vi "PRL DW Check Data CSG.vi"(11 "Data":csg[](array[numeric])) -> (3 "Bad Data?":bool[](array[boolean]))   [LabVIEW 2018, in "S3DK.lvlib" / "PMU Recorder Light.lvlib"]
uses:
  PMU Recorder Light.lvlib
  Setting Choice.ctl
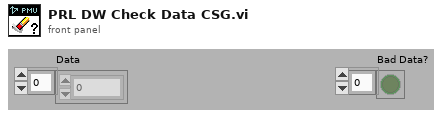
[diagram p1: front panel]
types:
  T1 = typedef "S3DK.lvlib/PMU Recorder Light.lvlib/Setting Choice.ctl" = enum16{"Analog Data Points Allowed Equals", "Complex Data Points Allowed Equals", "Seconds Before Reset After Wait for Config Fails", "Number of Live Buffer in Access Buffer ", "Number of Connection Attempts", "Live Data Buffer Size", "dt Tolerance", "Data Rate History", "ALL"}
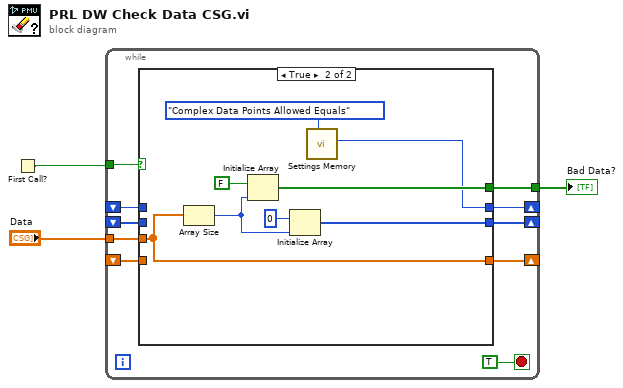
[diagram p0: block diagram]
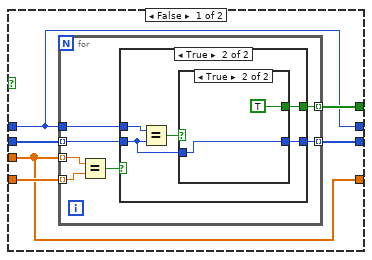
[diagram p2: hidden frame]
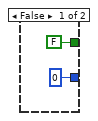
[diagram p3: hidden frame]
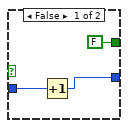
[diagram p4: hidden frame]
diagram:
  n1 = First Call?() -> (First Call?: T/F=w1:bool)
  n2 = while {
    tunnel: w1 -> [w13]
    tunnel: "Data" -> [w12]
    shift-right: [w10] -> _
    shift-left: _ -> [w7]
    shift-right: [w11] -> _
    shift-left: _ -> [w8]
    tunnel: [w9] -> w2
    shift-right: [w5] -> _
    shift-left: _ -> [w6]
    stop <- TRUE stop-if-true
    n3 = case shown="True" w13 {
      tunnel: w12 -> [w17 w44]
      tunnel: [w16 w45] -> w11
      tunnel: [w17 w44] -> w10
      tunnel: [w15 w41] -> w9
      tunnel: w8 -> [w19 _]
      tunnel: w7 -> [w18 _]
      tunnel: w6 -> [w14 _]
      tunnel: [w14 w39] -> w5
      frame False {
        n4 = for {
          tunnel: w19 -> [w23] mode=indexing
          tunnel: w17 -> [w25] mode=indexing
          tunnel: w18 -> [w26] mode=indexing
          tunnel: w14 -> [w22]
          tunnel: [w21] -> w16 mode=indexing
          tunnel: [w20] -> w15 mode=indexing
          n5 = Equal?(x=w25, y=w26) -> (x = y?=w24:bool)
          n6 = case shown="True" w24 {
            tunnel: w23 -> [_ w31]
            tunnel: w22 -> [_ w33]
            tunnel: [0 w30] -> w21
            tunnel: [FALSE w29] -> w20
            frame False {
            }
            frame True {
              n7 = Equal?(x=w33, y=w31) -> (x = y?=w32:bool)
              n8 = case shown="True" w32 {
                tunnel: w31 -> [w36 w38]
                tunnel: [w35 w38] -> w30
                tunnel: [FALSE TRUE] -> w29
                frame False {
                  n9 = Increment(x=w36) -> (x+1=w35:i32)
                }
                frame True {
                }
              }
            }
          }
        }
      }
      frame True {
        n10 = Array Size(array=w44) -> (size(s)=w43:i32)
        n11 = Initialize Array(FALSE, w43) -> (w41:bool[])
        n12 = Initialize Array(0, w43) -> (w45:i32[])
        n13 = call "Settings Memory.vi"("Setting Choice"=Setting_Choice."Complex Data Points Allowed Equals") -> ("Output Int32"=w39:i32)  [unwired: 8 in, 2 out]
      }
    }
  }
  "Bad Data?" <- w2
